vi "Print.vi"(10 "String":string, 11 "IPrinter In":refnum<class "IPrinter.lvclass">) -> (3 "IPrinter Out":refnum<class "IPrinter.lvclass">)   [LabVIEW 2018, in "IPrinter.lvclass"]
uses:
  IPrinter.lvclass
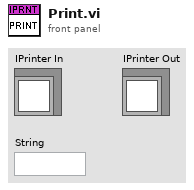
[diagram p1: front panel]
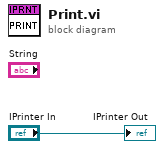
[diagram p0: block diagram]
diagram:
  "IPrinter Out" <- "IPrinter In"
